vi "Periodic Tasks.vi"(8 "error in":errorcluster) -> ()   [LabVIEW 2018]
doc: "This VI runs in parallel to other robot code. It can contain as many user-defined periodic loops as you need. These can carry out PID or other sorts of timed response."
uses:
  <vilib>/Rock Robotics/WPI/Utilities/WPI_GetSetVariantRefNum.vi
  Robot Global Data.vi
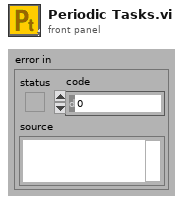
[diagram p1: front panel]
types:
  T1 = typedef "WPI_JoystickDevRef.ctl" = cluster{"Device":T2}
  T2 = typedef "WPI_JoystickDeviceEnum.ctl" = enum16{"USB 0", "USB 1", "USB 2", "USB 3", "USB 4", "USB 5"}
  T3 = cluster{"JoystickDevRef":T1, "JoystickDevRef":T1}
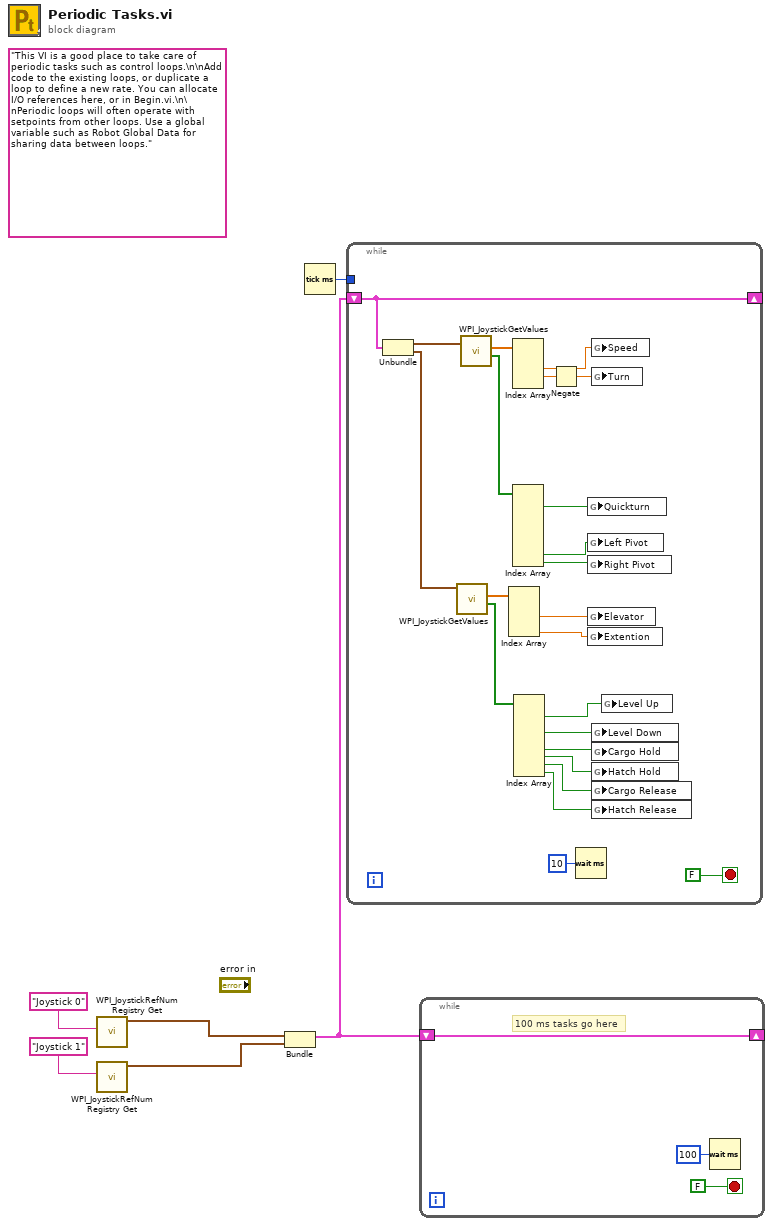
[diagram p0: block diagram]
diagram:
  (unwired) "This VI is a good place to take care of periodic tasks such as control loops.\n\nAdd code to the existing loops, or duplicate a loop to define a new rate. You can allocate I/O references here, or in Begin.vi.\n\nPeriodic loops will often operate with setpoints from other loops. Use a global variable such as Robot Global Data for sharing data between loops."
  n1 = call <vilib>:"WPI_JoystickRefNum Registry Get.vi"("refnum name"="Joystick 0") -> ("JoystickDevRef"=w3:T1)  [unwired: 1 in, 9 out]
  n2 = call <vilib>:"WPI_JoystickRefNum Registry Get.vi"("refnum name"="Joystick 1") -> ("JoystickDevRef"=w1:T1)  [unwired: 1 in, 9 out]
  n3 = Bundle("JoystickDevRef"=w3, "JoystickDevRef"=w1) -> (w2:T3)  [unwired: 1 in]
  n4 = Tick Count (ms)() -> (millisecond timer value=w5:u32)
  n5 = while {
    shift-right: [w19] -> _
    shift-left: w2 -> [w19]
    tunnel: w5 -> [_]
    stop <- FALSE stop-if-true
    n6 = Unbundle(w19) -> ("JoystickDevRef"=w18:T1, "JoystickDevRef"=w15:T1)
    n7 = call <vilib>:"WPI_JoystickGetValues.vi"("JoystickDevRef"=w15) -> ("Buttons"=w17:bool[], "Axes"=w16:dbl[])  [unwired: 6 in, 3 out]
    n8 = call <vilib>:"WPI_JoystickGetValues.vi"("JoystickDevRef"=w18) -> ("Buttons"=w25:bool[], "Axes"=w27:dbl[])  [unwired: 6 in, 3 out]
    n9 = Index Array(array=w16) -> (element #2=w8:dbl, element #4=w7:dbl)  [unwired: 4 in, 2 out]
    n10 = Index Array(array=w27) -> (element #2=w23:dbl, element #3=w22:dbl)  [unwired: 4 in, 2 out]
    n11 = Index Array(array=w25) -> (element #1=w24:bool, element #7=w21:bool, element #8=w20:bool)  [unwired: 8 in, 5 out]
    n12 = Index Array(array=w17) -> (element #1=w13:bool, element #3=w12:bool, element #5=w9:bool, element #6=w14:bool, element #7=w11:bool, element #8=w10:bool)  [unwired: 8 in, 2 out]
    n13 = Negate(x=w22) -> (-x=w26:dbl)
    n14 = Wait (ms)(milliseconds to wait=u32 10) -> ()  [unwired: 1 out]
    n15 = global write "Robot Global Data.vi" "Quickturn"(w24) -> ()
    n16 = global write "Robot Global Data.vi" "Left Pivot"(w21) -> ()
    n17 = global write "Robot Global Data.vi" "Right Pivot"(w20) -> ()
    n18 = global write "Robot Global Data.vi" "Elevator"(w8) -> ()
    n19 = global write "Robot Global Data.vi" "Extention"(w7) -> ()
    n20 = global write "Robot Global Data.vi" "Speed"(w23) -> ()
    n21 = global write "Robot Global Data.vi" "Turn"(w26) -> ()
    n22 = global write "Robot Global Data.vi" "Level Down"(w12) -> ()
    n23 = global write "Robot Global Data.vi" "Cargo Hold"(w9) -> ()
    n24 = global write "Robot Global Data.vi" "Hatch Hold"(w14) -> ()
    n25 = global write "Robot Global Data.vi" "Cargo Release"(w11) -> ()
    n26 = global write "Robot Global Data.vi" "Hatch Release"(w10) -> ()
    n27 = global write "Robot Global Data.vi" "Level Up"(w13) -> ()
  }
  n28 = while {
    shift-right: [w30] -> _
    shift-left: w2 -> [w30]
    stop <- FALSE stop-if-true
    # "100 ms tasks go here"
    n29 = Wait (ms)(milliseconds to wait=u32 100) -> ()  [unwired: 1 out]
  }
